vi "PAS CVT.vi"(8 "error in":errorcluster, 10 "refnum in":T1, 11 "Controller in":refnum<class "Controller.lvclass">) -> (0 "error out":errorcluster, 2 "refnum out":T1, 3 "Controller out":refnum<class "Controller.lvclass">)   [LabVIEW 2014, in "Controller.lvlib" / "Controller.lvclass"]
uses:
  Controller.lvclass
  <vilib>/Utility/config.llb/Config Data RefNum.ctl
  <vilib>/Utility/config.llb/Read Key (I32).vi
  <vilib>/Utility/config.llb/Read Key (Boolean).vi
  <vilib>/Utility/config.llb/Read Key (Double).vi
  <vilib>/Utility/config.llb/Read Key (String).vi
  <vilib>/Utility/config.llb/NI_LVConfig.lvlib
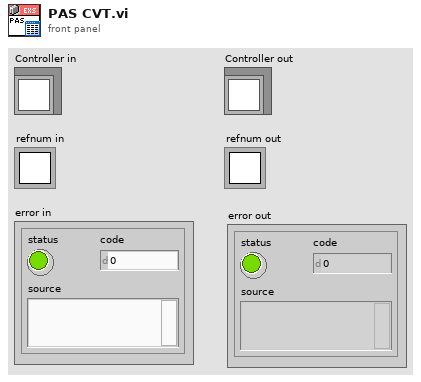
[diagram p1: front panel]
types:
  T1 = typedef "NI_LVConfig.lvlib/Config Data RefNum.ctl" = refnum<k1>
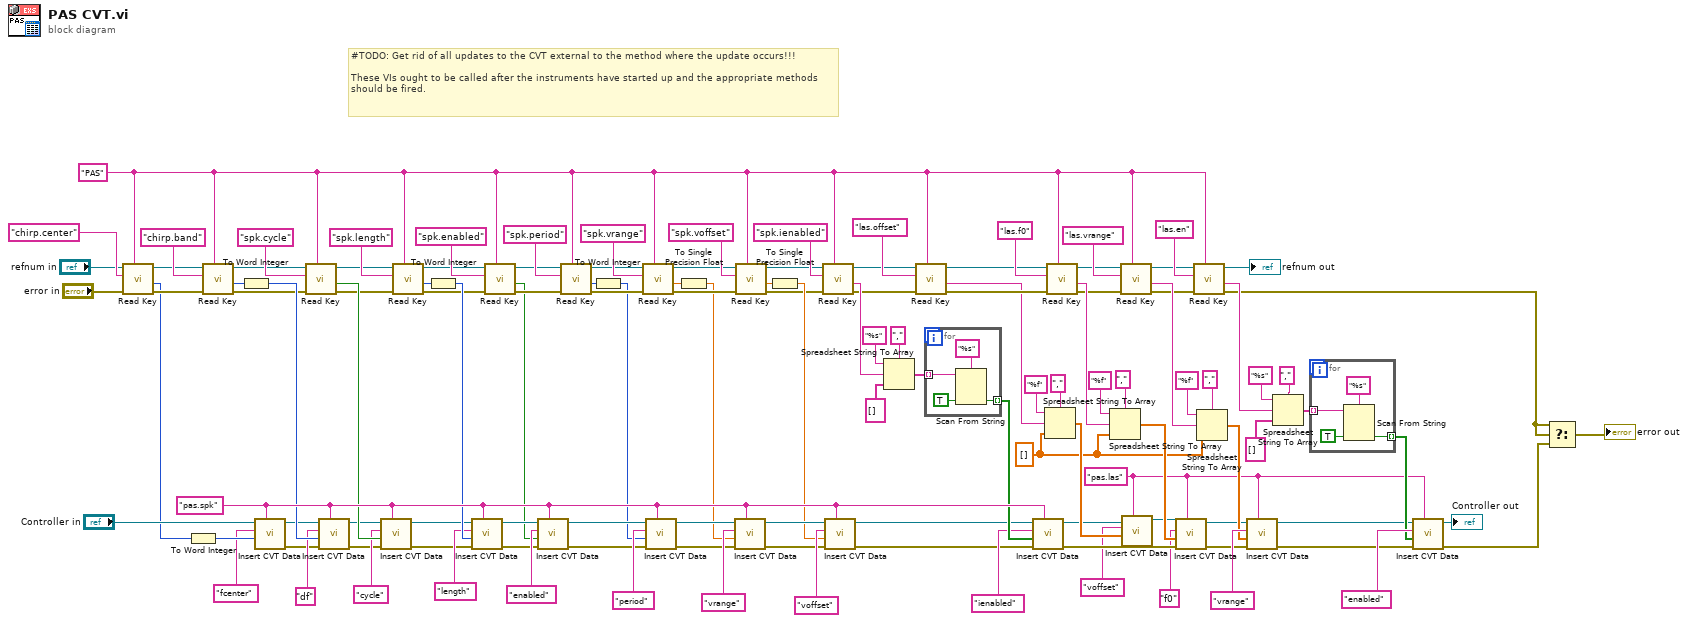
[diagram p0: block diagram]
diagram:
  w19 = "PAS" ("section")
  w8 = "pas.las" ("Group")
  w123 = "pas.spk" ("Group")
  w12 = sgl[] []
  # "#TODO: Get rid of all updates to the CVT external to the method where the update occurs!!!\n\nThese VIs ought to be called after the instruments have started up and the appropriate methods should be fired."
  n1 = call-poly <vilib>:"Read Key.vi"("section"=w19, "error in (no error)"="error in", "key"="chirp.center", "refnum"="refnum in") -> ("error out"=w39:errorcluster, "value"=w36:i32, "refnum out"=w37:T1)  [unwired: 4 in, 1 out]
  n2 = To Word Integer(number=w36) -> (16bit integer=w82:i16)
  n3 = call-poly <vilib>:"Read Key.vi"("section"=w19, "error in (no error)"=w39, "key"="chirp.band", "refnum"=w37) -> ("error out"=w42:errorcluster, "value"=w40:i32, "refnum out"=w41:T1)  [unwired: 4 in, 1 out]
  n4 = To Word Integer(number=w40) -> (16bit integer=w88:i16)
  n5 = call "Insert CVT Data.vi"("Group"=w123, "Data"=w82, "tag"="fcenter", "Controller in"="Controller in") -> ("error out"=w84:errorcluster, "Controller out"=w83:refnum<class "Controller.lvclass">)  [unwired: 6 in]
  n6 = call-poly <vilib>:"Read Key.vi"("section"=w19, "error in (no error)"=w42, "key"="spk.cycle", "refnum"=w41) -> ("error out"=w31:errorcluster, "value"=w90:bool, "refnum out"=w32:T1)  [unwired: 4 in, 1 out]
  n7 = call "Insert CVT Data.vi"("Group"=w123, "error in"=w84, "Data"=w88, "tag"="df", "Controller in"=w83) -> ("error out"=w85:errorcluster, "Controller out"=w86:refnum<class "Controller.lvclass">)  [unwired: 5 in]
  n8 = call "Insert CVT Data.vi"("Group"=w123, "error in"=w85, "Data"=w90, "tag"="cycle", "Controller in"=w86) -> ("error out"=w92:errorcluster, "Controller out"=w91:refnum<class "Controller.lvclass">)  [unwired: 5 in]
  n9 = call-poly <vilib>:"Read Key.vi"("section"=w19, "error in (no error)"=w31, "key"="spk.length", "refnum"=w32) -> ("error out"=w48:errorcluster, "value"=w46:i32, "refnum out"=w30:T1)  [unwired: 4 in, 1 out]
  n10 = To Word Integer(number=w46) -> (16bit integer=w94:i16)
  n11 = call "Insert CVT Data.vi"("Group"=w123, "error in"=w92, "Data"=w94, "tag"="length", "Controller in"=w91) -> ("error out"=w95:errorcluster, "Controller out"=w96:refnum<class "Controller.lvclass">)  [unwired: 5 in]
  n12 = call-poly <vilib>:"Read Key.vi"("section"=w19, "error in (no error)"=w48, "key"="spk.enabled", "refnum"=w30) -> ("error out"=w29:errorcluster, "value"=w2:bool, "refnum out"=w26:T1)  [unwired: 4 in, 1 out]
  n13 = call "Insert CVT Data.vi"("Group"=w123, "error in"=w95, "Data"=w2, "tag"="enabled", "Controller in"=w96) -> ("error out"=w98:errorcluster, "Controller out"=w99:refnum<class "Controller.lvclass">)  [unwired: 5 in]
  n14 = call-poly <vilib>:"Read Key.vi"("section"=w19, "error in (no error)"=w29, "key"="spk.period", "refnum"=w26) -> ("error out"=w28:errorcluster, "value"=w47:i32, "refnum out"=w25:T1)  [unwired: 4 in, 1 out]
  n15 = To Word Integer(number=w47) -> (16bit integer=w1:i16)
  n16 = call-poly <vilib>:"Read Key.vi"("section"=w19, "error in (no error)"=w28, "key"="spk.vrange", "refnum"=w25) -> ("error out"=w51:errorcluster, "value"=w53:dbl, "refnum out"=w50:T1)  [unwired: 4 in, 1 out]
  n17 = call "Insert CVT Data.vi"("Group"=w123, "error in"=w98, "Data"=w1, "tag"="period", "Controller in"=w99) -> ("error out"=w102:errorcluster, "Controller out"=w101:refnum<class "Controller.lvclass">)  [unwired: 5 in]
  n18 = To Single Precision Float(number=w53) -> (single precision float=w23:sgl)
  n19 = call "Insert CVT Data.vi"("Group"=w123, "error in"=w102, "Data"=w23, "tag"="vrange", "Controller in"=w101) -> ("error out"=w105:errorcluster, "Controller out"=w104:refnum<class "Controller.lvclass">)  [unwired: 5 in]
  n20 = call-poly <vilib>:"Read Key.vi"("section"=w19, "error in (no error)"=w51, "key"="spk.voffset", "refnum"=w50) -> ("error out"=w15:errorcluster, "value"=w52:dbl, "refnum out"=w16:T1)  [unwired: 4 in, 1 out]
  n21 = To Single Precision Float(number=w52) -> (single precision float=w24:sgl)
  n22 = call-poly <vilib>:"Read Key.vi"("section"=w19, "error in (no error)"=w15, "key"="spk.ienabled", "refnum"=w16) -> ("error out"=w21:errorcluster, "value"=w79:string, "refnum out"=w22:T1)  [unwired: 4 in, 1 out]
  n23 = call "Insert CVT Data.vi"("Group"=w123, "error in"=w105, "Data"=w24, "tag"="voffset" ("key"), "Controller in"=w104) -> ("error out"=w118:errorcluster, "Controller out"=w117:refnum<class "Controller.lvclass">)  [unwired: 5 in]
  n24 = Spreadsheet String To Array(delimiter (Tab)=",", format string="%s", spreadsheet string=w79, array type (2D Dbl)=string[] []) -> (array=w75:string[])
  n25 = call-poly <vilib>:"Read Key.vi"("section"=w19, "error in (no error)"=w21, "key"="las.offset", "refnum"=w22) -> ("error out"=w64:errorcluster, "value"=w27:string, "refnum out"=w63:T1)  [unwired: 4 in, 1 out]
  n26 = for {
    tunnel: w75 -> [w127] mode=indexing
    tunnel: [w124] -> w121 mode=indexing
    n27 = Scan From String(format string="%s", input string=w127, default 1=TRUE) -> (output 1=w124:bool)  [unwired: 2 in, 3 out]
  }
  n28 = call "Insert CVT Data.vi"("Group"=w123, "error in"=w118, "Data"=w121, "tag"="ienabled" ("key"), "Controller in"=w117) -> ("error out"=w119:errorcluster, "Controller out"=w7:refnum<class "Controller.lvclass">)  [unwired: 5 in]
  n29 = Spreadsheet String To Array(delimiter (Tab)=",", format string="%f", spreadsheet string=w27, array type (2D Dbl)=w12) -> (array=w114:sgl[])
  n30 = call-poly <vilib>:"Read Key.vi"("section"=w19, "error in (no error)"=w64, "key"="las.f0", "refnum"=w63) -> ("error out"=w13:errorcluster, "value"=w20:string, "refnum out"=w14:T1)  [unwired: 4 in, 1 out]
  n31 = Spreadsheet String To Array(delimiter (Tab)=",", format string="%f", spreadsheet string=w20, array type (2D Dbl)=w12) -> (array=w108:sgl[])
  n32 = call-poly <vilib>:"Read Key.vi"("section"=w19, "error in (no error)"=w13, "key"="las.vrange", "refnum"=w14) -> ("error out"=w17:errorcluster, "value"=w57:string, "refnum out"=w18:T1)  [unwired: 4 in, 1 out]
  n33 = call "Insert CVT Data.vi"("Group"=w8, "Data"=w114, "tag"="voffset" ("Tag Name"), "Controller in"=w7) -> ("Controller out"=w6:refnum<class "Controller.lvclass">)  [unwired: 6 in, 1 out]
  n34 = call "Insert CVT Data.vi"("Group"=w8, "error in"=w119, "Data"=w108, "tag"="f0", "Controller in"=w6) -> ("error out"=w110:errorcluster, "Controller out"=w109:refnum<class "Controller.lvclass">)  [unwired: 5 in]
  n35 = call-poly <vilib>:"Read Key.vi"("section"=w19, "error in (no error)"=w17, "key"="las.en", "refnum"=w18) -> ("error out"=w5:errorcluster, "value"=w72:string, "refnum out"=→"refnum out":T1)  [unwired: 4 in, 1 out]
  n36 = Spreadsheet String To Array(delimiter (Tab)=",", format string="%f", spreadsheet string=w57, array type (2D Dbl)=w12) -> (array=w111:sgl[])
  n37 = call "Insert CVT Data.vi"("Group"=w8, "error in"=w110, "Data"=w111, "tag"="vrange" ("key"), "Controller in"=w109) -> ("error out"=w9:errorcluster, "Controller out"=w10:refnum<class "Controller.lvclass">)  [unwired: 5 in]
  n38 = Spreadsheet String To Array(delimiter (Tab)=",", format string="%s", spreadsheet string=w72, array type (2D Dbl)=string[] []) -> (array=w71:string[])
  n39 = for {
    tunnel: w71 -> [w131] mode=indexing
    tunnel: [w128] -> w115 mode=indexing
    n40 = Scan From String(format string="%s", input string=w131, default 1=TRUE) -> (output 1=w128:bool)  [unwired: 2 in, 3 out]
  }
  n41 = call "Insert CVT Data.vi"("Group"=w8, "error in"=w9, "Data"=w115, "tag"="enabled" ("Tag Name"), "Controller in"=w10) -> ("error out"=w4:errorcluster, "Controller out"=→"Controller out":refnum<class "Controller.lvclass">)  [unwired: 5 in]
  n42 = Select(t=w5, s=w5, f=w4) -> (s? t:f=→"error out":errorcluster)
